vi "Splash Screen (RoboSys).vi"(8 "Error In":errorcluster) -> ()   [LabVIEW 2014]
uses:
  SubVI/State/SubVI/Set Splash Screen State.vi
  SubVI/State/SubVI/Get Splash Screen State.vi
  System.Windows.Forms
  System.Drawing
panel:
  in  "PictureBox":refnum<k24>(container)
  out "Error Out":errorcluster
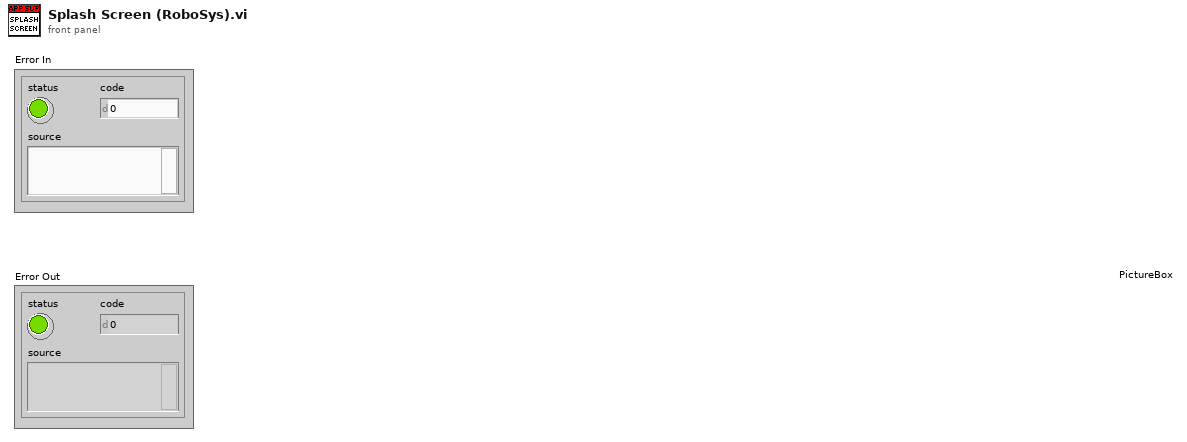
[diagram p1: front panel]
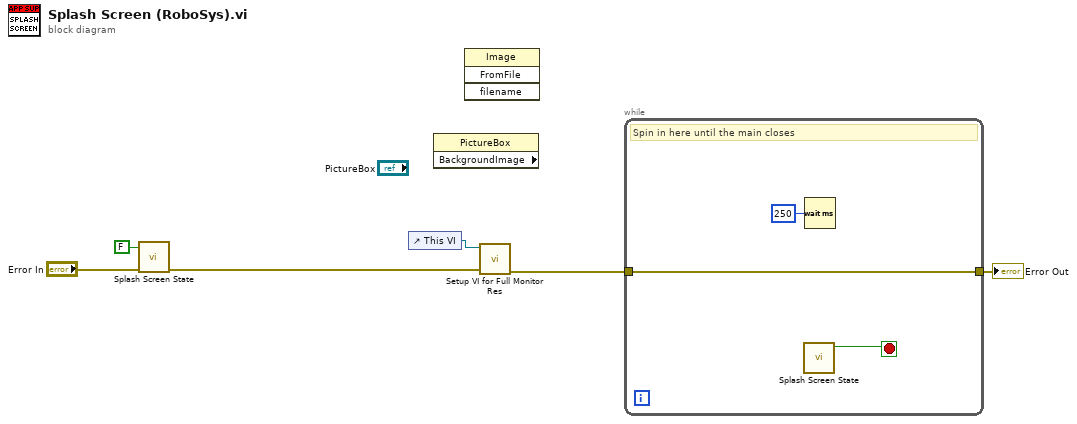
[diagram p0: block diagram]
diagram:
  n1 = call-poly "Splash Screen State.vi"("Error In"="Error In", "Close Splash Screen"=FALSE) -> ("Error Out"=w3:errorcluster)  [unwired: 9 in]
  n2 = control-ref of="This VI"() -> (w6:refnum<vi>)
  n3 = property class="PictureBox" props=["BackgroundImage"]() -> ()  [unwired: 2 in, 3 out]
  n4 = invoke class="Image" method="FromFile"() -> ()  [unwired: 4 in, 4 out]
  n5 = call "Setup VI for Full Monitor Res.vi"("Error In"=w3, "This VI"=w6) -> ("Error Out"=w5:errorcluster)  [unwired: 8 in, 1 out]
  n6 = while {
    tunnel: w5 -> [w8]
    tunnel: [w8] -> w4
    stop <- w7 stop-if-true
    # "Spin in here until the main closes"
    n7 = call-poly "Splash Screen State.vi"() -> ("Close Splash Screen Out"=w7:bool)  [unwired: 10 in, 1 out]
    n8 = Wait (ms)(milliseconds to wait=u32 250) -> ()  [unwired: 1 out]
  }
  "Error Out" <- w4
